vi "Single motor operation(Joint mode).vi"() -> ()   [LabVIEW 2016]
uses:
  <instrlib>/Dynamixel Motor/Public/Motor Operation/Low Level/Baud Setting.ctl
  <instrlib>/Dynamixel Motor/Dynamixel Motor.lvlib
panel:
  in  "Motor ID (0)":u8
  in  "정지":bool
  in  "Goal Position (180 deg)":dbl=180.0
  in  "Baud rate (57600 bps)":T1=34 items=["1,000,000 bps"=1, "500,000 bps"=3, "400,000 bps"=4, "250,000 bps"=7, "200,000 bps"=9, "115200 bps"=16, "57600 bps"=34, "19200 bps"=103, "9600 bps"=207]
  in  "VISA resource name":refnum<visa-resource-name>
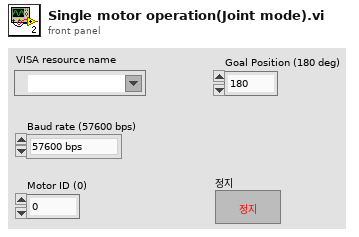
[diagram p1: front panel]
types:
  T1 = typedef "Dynamixel Motor.lvlib/Baud Setting.ctl" = u8
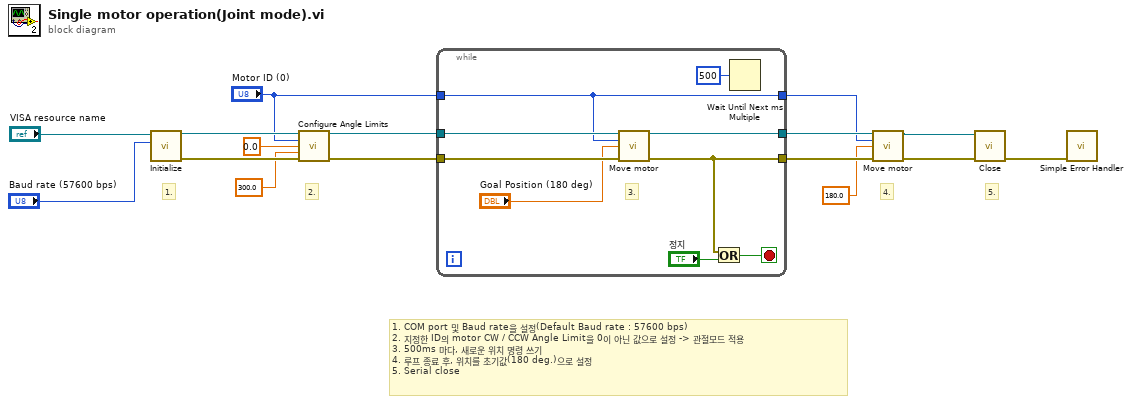
[diagram p0: block diagram]
diagram:
  # "5."
  # "1. COM port 및 Baud rate을 설정(Default Baud rate : 57600 bps)\n2. 지정한 ID의 motor CW / CCW Angle Limit을 0이 아닌 값으로 설정 -> 관절모드 적용\n3. 500ms 마다, 새로운 위치 명령 쓰기\n4. 루프 종료 후, 위치를 초기값(180 deg.)으로 설정\n5. Serial close"
  # "2."
  # "4."
  # "1."
  n1 = call <instrlib>:"Initialize.vi"("Baud rate (57600 bps)"="Baud rate (57600 bps)", "VISA resource name"="VISA resource name") -> ("error out"=w15:errorcluster, "VISA resource name out"=w16:refnum<visa-resource-name>)  [unwired: 8 in]
  n2 = call <instrlib>:"Configure Angle Limits.vi"("VISA resource name"=w16, "Motor ID (0)"="Motor ID (0)", "Clockwise Angle Limit (0 deg)"=0.0, "Counter-Clockwise Angle Limit (300 deg)"=300.0, "error in (no error)"=w15) -> ("VISA resource name out"=w11:refnum<visa-resource-name>, "error out"=w10:errorcluster)  [unwired: 9 in]
  n3 = while {
    tunnel: "Motor ID (0)" -> [w20]
    tunnel: [w20] -> w2
    tunnel: w11 -> [w25]
    tunnel: [w23] -> w6
    tunnel: w10 -> [w24]
    tunnel: [w19] -> w3
    stop <- w17 stop-if-true
    # "3."
    n4 = call <instrlib>:"Move motor.vi"("VISA resource name"=w25, "Motor ID (0)"=w20, "Goal Position (180 deg)"="Goal Position (180 deg)", "error in (no error)"=w24) -> ("VISA resource name out"=w23:refnum<visa-resource-name>, "error out"=w19:errorcluster)  [unwired: 10 in]
    n5 = Or(x=w19, y="정지") -> (x .or. y?=w17:bool)
    n6 = Wait Until Next ms Multiple(millisecond multiple=u32 500 ("ms 배수")) -> ()  [unwired: 1 out]
  }
  n7 = call <instrlib>:"Move motor.vi"("VISA resource name"=w6, "Motor ID (0)"=w2, "Goal Position (180 deg)"=180.0, "error in (no error)"=w3) -> ("VISA resource name out"=w5:refnum<visa-resource-name>, "error out"=w4:errorcluster)  [unwired: 10 in]
  n8 = call <instrlib>:"Close.vi"("error in (no error)"=w4, "VISA resource name"=w5) -> ("error out"=w14:errorcluster)  [unwired: 9 in]
  n9 = call <vilib>:"Simple Error Handler.vi"("error in (no error)"=w14) -> ()  [unwired: 4 in, 5 out]
